vi "LVCAM Receive.vi"(11 "LVCAM Receive in":refnum<class "LVCAM Receive.lvclass">) -> (0 "error out":errorcluster, 2 "Msg":refnum<class "Msg.lvclass">)   [LabVIEW 2021, in "LVCAM.lvlib" / "LVCAM Receive.lvclass"]
uses:
  LVCAM Receive.lvclass
  Msg/Msg.lvclass
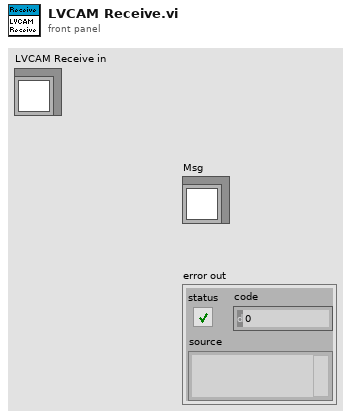
[diagram p1: front panel]
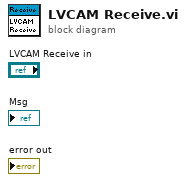
[diagram p0: block diagram]
diagram:
